vi "PV Digiline Data.vi"(8 "error in (no error)":errorcluster, 9 "DigiLine-Cluster":T1={"Parameter"=0, "Parameter\nread only<->describe"=FALSE, "Correction factor\n(0,20 - 9,90) "=1.0, "Pressure set point (mbar)\n0 ==> ur (p<1,0e-4 mbar)\n1 - 2050 mbar"=0} {"Pressure set point (mbar)\n0 ==> ur (p<1,0e-4 mbar)\n1 - 2050 mbar" min=0 max=2050 step=1; "Correction factor\n(0,20 - 9,90)" min=0.2 max=9.9 step=0.01 format="%.2f"; "Parameter" items=[" Pressure  [mbar]", " Correction factor 1", " Correction factor 2 (Bayard Albert)", " Actual error code (read only)", " Software version Transmitter  (read only)", " Unit type Transmitter (read only)"]}, 10 "Adress of unit":u16=1 max=999 step=1, 11 "VISA session":refnum<visa-resource-name>) -> (0 "error out":errorcluster, 2 "response (data)":string, 3 "dup VISA session":refnum<visa-resource-name>)   [LabVIEW 2024, in "Pfeiffer Vacuum.lvlib"]
doc: "There are 6 parameters available, only one of which can be enabled at a time. \n\n0 - Pressure [mbar] (default)\n1 - Correction factor 1 \n2 - Correction factor 2 (Bayard Albert only)\n3 - Actual error code (read only)\n4 - Software version Transmitter (read only)\n5 - Unit type Transmitter (read only)\n\nNote: The 2 controls right of this one will set the appropriate values for the selected parameter. Any settings for an parameter that is not selected will be ignored. If a value is out of range, it will be changed to either the upper or the lower limit of the range."
uses:
  <instrlib>/Pfeiffer Vacuum/Pfeiffer Vacuum.lvlib
  <instrlib>/Pfeiffer Vacuum/Public/DigiLine/PV Digiline - Cluster.ctl
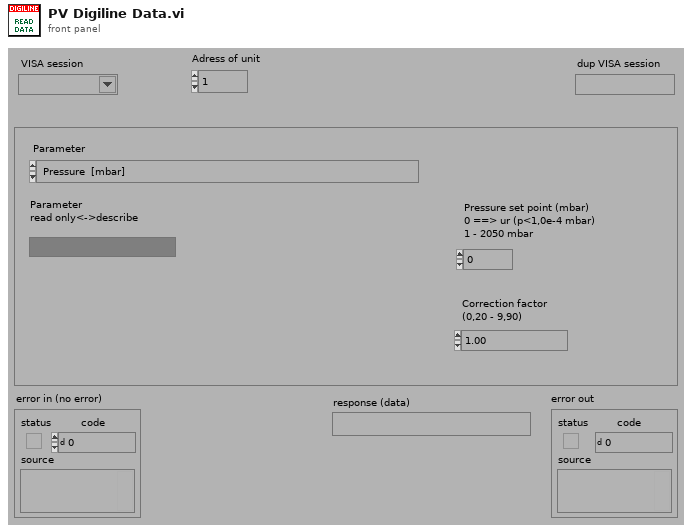
[diagram p1: front panel]
types:
  T1 = typedef "Pfeiffer Vacuum.lvlib/PV Digiline - Cluster.ctl" = cluster{"Parameter":u16, "Parameter\nread only<->describe":bool, "Correction factor\n(0,20 - 9,90) ":sgl, "Pressure set point (mbar)\n0 ==> ur (p<1,0e-4 mbar)\n1 - 2050 mbar":i16}
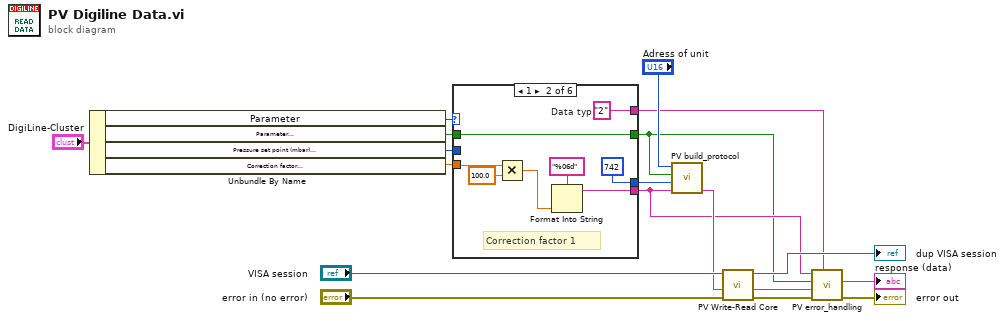
[diagram p0: block diagram]
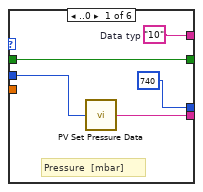
[diagram p2: hidden frame]
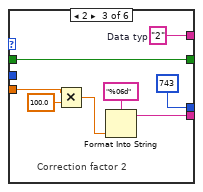
[diagram p3: hidden frame]
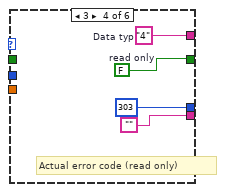
[diagram p4: hidden frame]
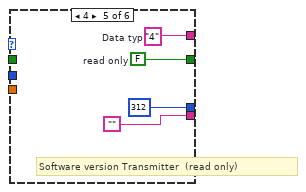
[diagram p5: hidden frame]
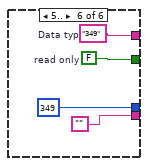
[diagram p6: hidden frame]
diagram:
  n1 = Unbundle By Name("DigiLine-Cluster") -> ("Parameter"=w15:u16, "Parameter\nread only<->describe"=w14:bool, "Pressure set point (mbar)\n0 ==> ur (p<1,0e-4 mbar)\n1 - 2050 mbar"=w12:i16, "Correction factor\n(0,20 - 9,90)"=w1:sgl)
  n2 = case shown="1" w15 {
    tunnel: [u16 740 ("Parameter-number") u16 742 ("Parameter-number") u16 743 ("Parameter-number") u16 303 ("Parameter-number") u16 312 ("Parameter-number") u16 349 ("Parameter-number")] -> w17
    tunnel: [w21 w24 w32 "" "" ""] -> w4
    tunnel: [w22 w30 w38 w42 w45 w51] -> w3
    tunnel: w14 -> [w22 w30 w38 _ _ _]
    tunnel: w12 -> [w20 _ _ _ _ _]
    tunnel: w1 -> [_ w27 w34 _ _ _]
    tunnel: [w19 w29 w37 w40 w44 w48] -> w5
    frame ..0 {
      w19 = "10"  # Data typ
      # "Pressure  [mbar]"
      n3 = call <instrlib>:"PV Set Pressure Data.vi"("Pressure (mbar)\n0 ==> ur (<1,0e-4mbar)\n1 - 2050 mbar"=w20) -> ("Output"=w21:string)
    }
    frame 1 {
      w29 = "2"  # Data typ
      # "Correction factor 1"
      n4 = Multiply(x=w27, y=100.0) -> (x*y=w25:dbl)
      n5 = Format Into String(format string="%06d" ("Format-String"), w25) -> (resulting string=w24:string)  [unwired: 2 in, 1 out]
    }
    frame 2 {
      w37 = "2"  # Data typ
      # "Correction factor 2"
      n6 = Multiply(x=w34, y=100.0) -> (x*y=w33:dbl)
      n7 = Format Into String(format string="%06d" ("Format-String"), w33) -> (resulting string=w32:string)  [unwired: 2 in, 1 out]
    }
    frame 3 {
      w40 = "4"  # Data typ
      w42 = FALSE  # read only
      # "Actual error code (read only)"
    }
    frame 4 {
      w44 = "4"  # Data typ
      w45 = FALSE  # read only
      # "Software version Transmitter  (read only)"
    }
    frame 5.. {
      w48 = "349"  # Data typ
      w51 = FALSE  # read only
    }
  }
  n8 = call <instrlib>:"PV build_protocol.vi"("Data"=w4, "Parameter-number"=w17, "parameter\nread<->describe"=w3, "Adress"="Adress of unit") -> ("output"=w9:string)  [unwired: 3 in]
  n9 = call <instrlib>:"PV Write-Read Core.vi"("error in"="error in (no error)", "Write data in"=w9, "VISA session"="VISA session") -> ("error out"=w6:errorcluster, "response (data) out"=w7:string, "dup VISA session"=→"dup VISA session":refnum<visa-resource-name>)  [unwired: 2 in]
  n10 = call <instrlib>:"PV error_handling.vi"("Data Typ in"=w5, "error in"=w6, "response (data) in"=w7, "Parameter\nread only<->describe"=w3, "data in"=w4) -> ("error out"=→"error out":errorcluster, "Data out"=→"response (data)":string)  [unwired: 4 in, 1 out]
